vi "mtg reader - fill table with filenames.vi"(11 "short file names":string[](array[string])) -> (3 "session files table":string[][](array[string]))   [LabVIEW 2025]
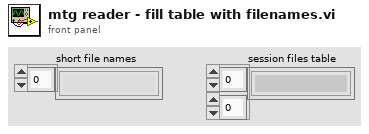
[diagram p1: front panel]
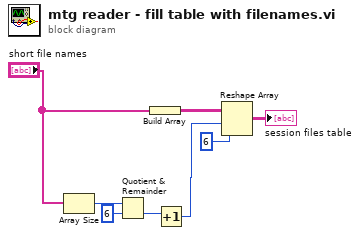
[diagram p0: block diagram]
diagram:
  n1 = Array Size(array="short file names") -> (size(s)=w5:i32)
  n2 = Quotient & Remainder(x=w5, y=6) -> (floor(x/y)=w7:i32)  [unwired: 1 out]
  n3 = Build Array("short file names") -> (w1:string[][])
  n4 = Increment(x=w7) -> (x+1=w8:i32)
  n5 = Reshape Array(w1, w8, 6 ("dimension size")) -> (→"session files table":string[][])
